vi "Load Plugins.vi"(8 "error in (no error)":errorcluster, 11 "User Interface References":T1) -> (0 "error out":errorcluster, 2 "Array of Plugins Out":refnum<class "Generic Plugin.lvclass">[](array[class]), 3 "User Interface References Out":T1)   [LabVIEW 2011]
uses:
  Menu Buttons_old/Menu Button XControl/Menu Button XControl.xctl
  Parent Plugin Definition/Plugin Template/Generic Plugin.lvclass
  Framework SubVIs/Plugin Handler/Plugin Command Manager/Plugin Load from Disk/Plugin Load from Disk.lvclass
  <vilib>/Utility/config.llb/NI_LVConfig.lvlib
  <vilib>/Utility/config.llb/Read Key (Path).vi
  Sliding Menu Type Definitions/User Interface Type Definitions.ctl
  <vilib>/Utility/config.llb/Config Data RefNum.ctl
  Sliding Menu Type Definitions/UI Picture Containers.ctl
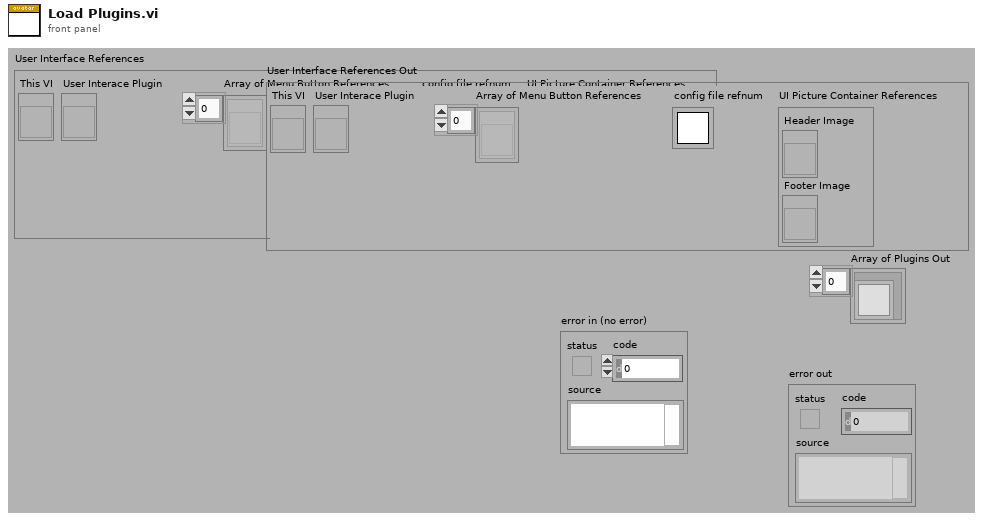
[diagram p1: front panel]
types:
  T1 = typedef "Sliding Menu Control.lvlib/User Interface Type Definitions.ctl" = cluster{"This VI":refnum<vi>, "User Interace Plugin":refnum<vi>, "Array of Menu Button References":refnum<vi>[], "config file refnum":T2, "UI Picture Container References":T3}
  T2 = typedef "NI_LVConfig.lvlib/Config Data RefNum.ctl" = refnum<k1>
  T3 = typedef "UI Picture Containers.ctl" = cluster{"Header Image":refnum<vi>, "Footer Image":refnum<vi>}
  T4 = enum16{"Initialize Test Data", "Get Entire Array", "Store Plugins"}
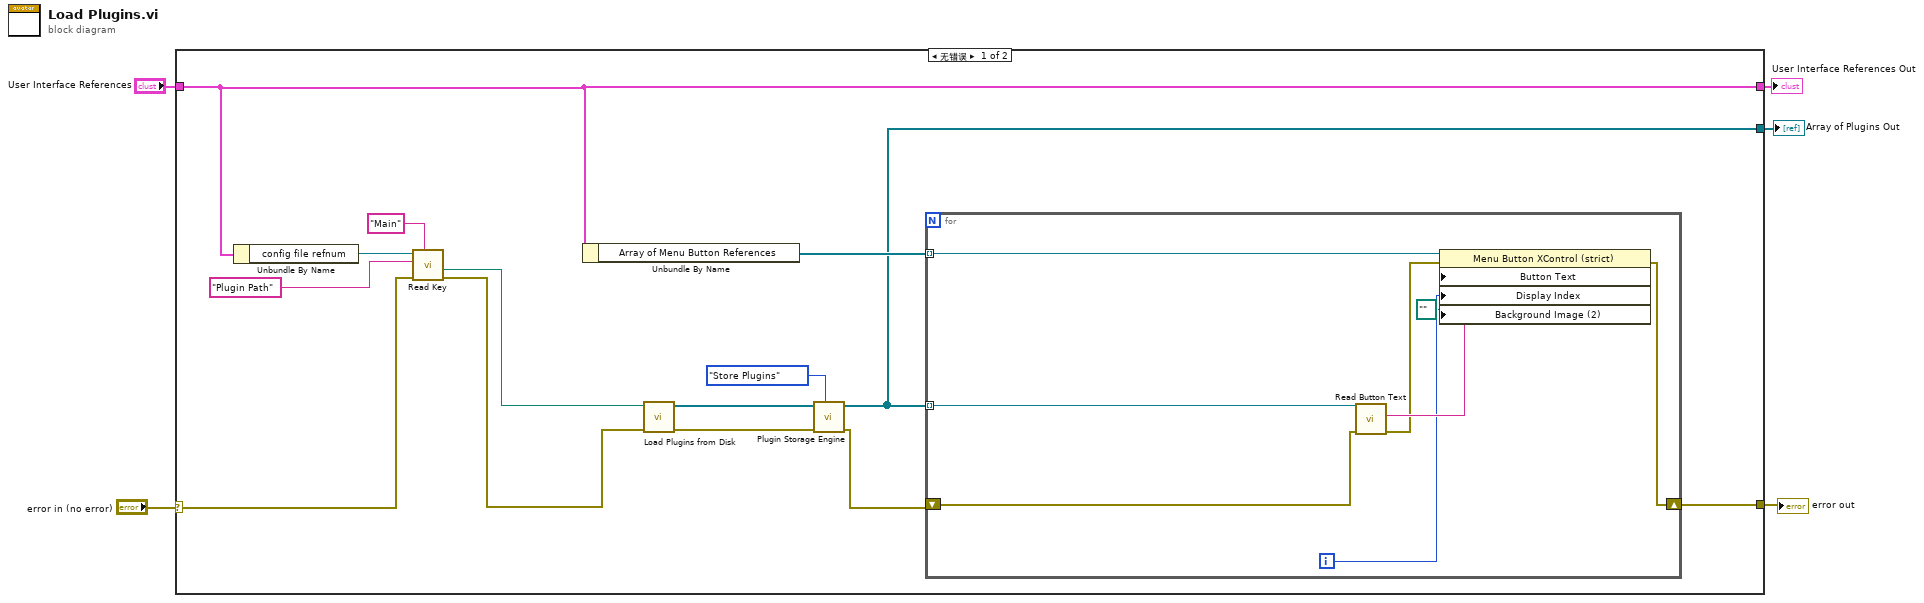
[diagram p0: block diagram]
diagram:
  n1 = case shown="无错误" "error in (no error)" {
    selector: "error in (no error)" -> [w9 w29]
    tunnel: [w16 w29] -> w5
    tunnel: [w13 w28] -> w2
    tunnel: "User Interface References" -> [w13 w28]
    tunnel: [w6 _] -> w1
    frame No Error {
      n2 = Unbundle By Name(w13) -> ("config file refnum"=w12:T2)
      n3 = call-poly <vilib>:"Read Key.vi"("section"="Main", "error in (no error)"=w9, "key"="Plugin Path", "refnum"=w12) -> ("error out"=w10:errorcluster, "value"=w11:path)  [unwired: 4 in, 2 out]
      n4 = Unbundle By Name(w13) -> ("Array of Menu Button References"=w19:refnum<vi>[])
      n5 = call "Load Plugins from Disk.vi"("error in (no error)"=w10, "Plugin Location on Disk"=w11) -> ("error out"=w14:errorcluster, "Array of Plugins"=w15:refnum<class "Generic Plugin.lvclass">[])  [unwired: 8 in]
      n6 = call "Plugin Storage Engine.vi"("Actions"=T4."Store Plugins", "error in (no error)"=w14, "Array of Plugins"=w15) -> ("error out"=w18:errorcluster, "Array of Plugins Out"=w6:refnum<class "Generic Plugin.lvclass">[])  [unwired: 7 in]
      n7 = for {
        tunnel: w19 -> [w27] mode=indexing
        shift-right: [w26] -> w16
        shift-left: w18 -> [w22]
        tunnel: w6 -> [w25] mode=indexing
        i -> [w21]
        n8 = call-dynamic "Read Button Text.vi"("error in (no error)"=w22, "Generic Plugin in"=w25) -> ("error out"=w23:errorcluster, "Button Text"=w24:string)  [unwired: 7 in, 1 out]
        n9 = property class="Menu Button XControl (strict)"(reference=w27, error in=w23, "Button Text"=w24, "Display Index"=w21, "Background Image (2)"=path "" ("Background Image")) -> (error out=w26:errorcluster)  [unwired: 1 out]
      }
    }
    frame Error {
    }
  }
  "error out" <- w5
  "User Interface References Out" <- w2
  "Array of Plugins Out" <- w1
